vi "Enum Data Patch.vi"(7 "Ref":variant, 8 "error in (no error)":errorcluster, 11 "data in":variant) -> (0 "error out":errorcluster, 3 "data out":variant)   [LabVIEW 2017]
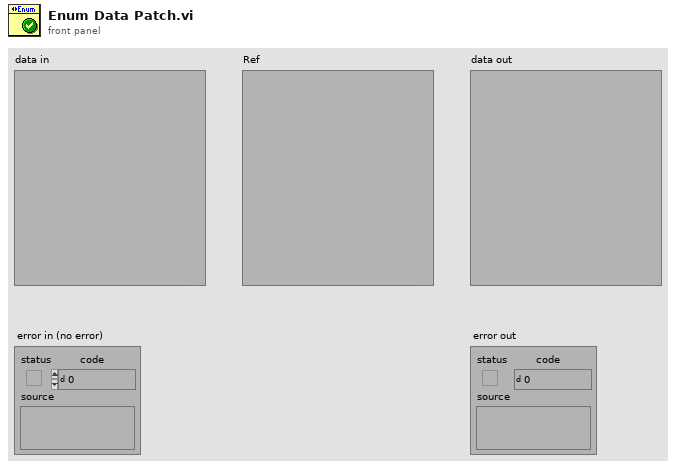
[diagram p1: front panel]
types:
  T1 = typedef "Type Descriptor Enumeration__ogtk.ctl" = enum8{"<Null>", "I8", "I16", "I32", "I64", "U8", "U16", "U32", "U64", "SGL", "DBL", "EXT", "CSG", "CDB", "CXT", "0x0F", "0x10", "0x11", "0x12", "0x13", "0x14", "Enum U8", "Enum U16", "Enum U32", "Enum U64", "SGL PQ", "DBL PQ", "EXT PQ", "CSG PQ", "CDB PQ", "CXT PQ", "0x1F", "0x20", "Boolean", "0x22", "0x23", "0x24", "0x25", "0x26", "0x27", "0x28", "0x29", "0x2A", "0x2B", "0x2C", "0x2D", "0x2E", "0x2F", "String", "0x31", "Path", "Pict", "0x34", "0x35", "0x36", "DAQ", "0x38", "0x39", "0x3A", "0x3B", "0x3C", "0x3D", "0x3E", "0x3F", "Array", "0x41", "0x42", "0x43", "0x44", "0x45", "0x46", "0x47", "0x48", "0x49", "0x4A", "0x4B", "0x4C", "0x4D", "0x4E", "0x4F", "Cluster", "0x51", "0x52", "Variant", "Waveform", "0x55", "0x56", "0x57", "0x58", "0x59", "0x5A", "0x5B", "0x5C", "0x5D", "0x5E", "0x5F", "0x60", "0x61", "0x62", "0x63", "0x64", "0x65", "0x66", "0x67", "0x68", "0x69", "0x6A", "0x6B", "0x6C", "0x6D", "0x6E", "0x6F", "Refnum"}
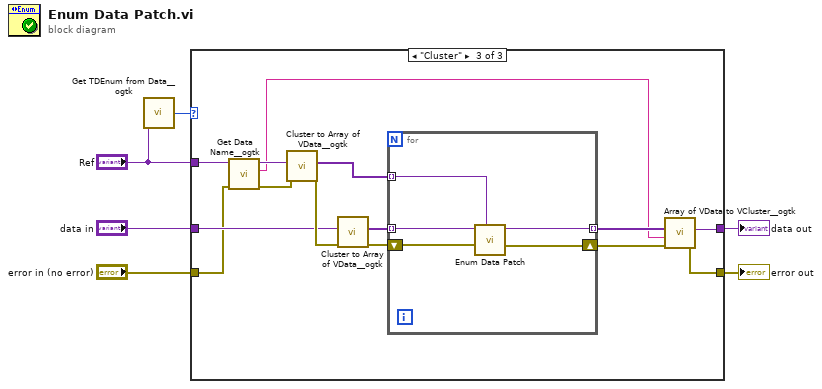
[diagram p0: block diagram]
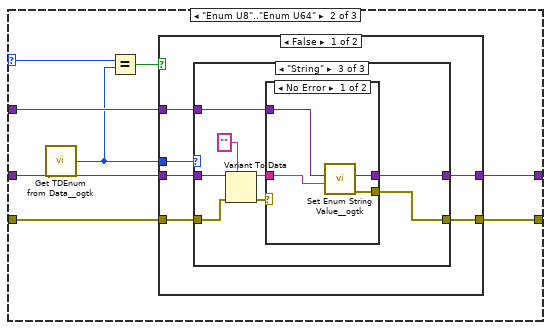
[diagram p3: hidden frame]
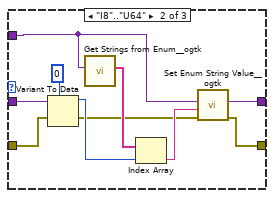
[diagram p5: hidden frame]
diagram:
  n1 = call <userlib>:"Get TDEnum from Data__ogtk.vi"("Data"="Ref") -> ("Type Descriptor Enumeration"=w6:T1)  [unwired: 4 in]
  n2 = case shown="\"Cluster\"" w6 {
    selector: w6 -> [_ w16 _]
    tunnel: [w8 w13 w63] -> w5
    tunnel: "data in" -> [w8 w10 w53]
    tunnel: "error in (no error)" -> [w7 w11 w52]
    tunnel: [w7 w12 w58] -> w2
    tunnel: "Ref" -> [_ w14 w55]
    frame Default {
    }
    frame "Enum U8".."Enum U64" {
      n3 = call <userlib>:"Get TDEnum from Data__ogtk.vi"("Data"=w10) -> ("Type Descriptor Enumeration"=w9:T1)  [unwired: 4 in]
      n4 = Equal?(x=w16, y=w9) -> (x = y?=w15:bool)
      n5 = case shown="False" w15 {
        tunnel: w14 -> [w21 _]
        tunnel: [w19 w48] -> w13
        tunnel: [w18 w49] -> w12
        tunnel: w11 -> [w17 w49]
        tunnel: w10 -> [w20 w48]
        tunnel: w9 -> [w22 _]
        frame False {
          n6 = case shown="\"String\"" w22 {
            tunnel: w21 -> [w24 w32 w41]
            tunnel: w20 -> [_ w34 w40]
            tunnel: [w24 w28 w42] -> w19
            tunnel: [w23 w26 w37] -> w18
            tunnel: w17 -> [w23 w25 w36]
            frame "<Null>", Default {
            }
            frame "I8".."U64" {
              n7 = Variant To Data(error in=w25, type=i64 0, Variant=w34) -> (data=w30:i64, error out=w27:errorcluster)
              n8 = call <userlib>:"Get Strings from Enum__ogtk.vi"("Enum"=w32) -> ("Enum Strings"=w31:string[])  [unwired: 7 in, 3 out]
              n9 = Index Array(array=w31, index=w30) -> (element=w29:string)
              n10 = call <userlib>:"Set Enum String Value__ogtk.vi"("error in (no error)"=w27, "String Value"=w29, "Default Enum Value"=w32) -> ("error out"=w26:errorcluster, "Enum"=w28:variant)  [unwired: 7 in]
            }
            frame "String" {
              n11 = Variant To Data(error in=w36, type="", Variant=w40) -> (data=w38:string, error out=w35:errorcluster)
              n12 = case shown="No Error" w35 {
                tunnel: [w46 w47] -> w42
                tunnel: w41 -> [w45 w47]
                tunnel: w38 -> [w44 _]
                tunnel: [w43 _] -> w37
                frame No Error {
                  n13 = call <userlib>:"Set Enum String Value__ogtk.vi"("String Value"=w44, "Default Enum Value"=w45) -> ("error out"=w43:errorcluster, "Enum"=w46:variant)  [unwired: 8 in]
                }
                frame Error {
                }
              }
            }
          }
        }
        frame True {
        }
      }
    }
    frame "Cluster" {
      n14 = call <userlib>:"Get Data Name__ogtk.vi"("error in (no error)"=w52, "Data"=w55) -> ("error out"=w51:errorcluster, "Data Name"=w50:string, "Data dup"=w54:variant)  [unwired: 7 in]
      n15 = call <userlib>:"Cluster to Array of VData__ogtk.vi"("error in (no error)"=w51, "Cluster"=w54) -> ("error out"=w56:errorcluster, "Array of VData"=w57:variant[])  [unwired: 8 in]
      n16 = call <userlib>:"Cluster to Array of VData__ogtk.vi"("error in (no error)"=w56, "Cluster"=w53) -> ("error out"=w60:errorcluster, "Array of VData"=w62:variant[])  [unwired: 8 in]
      n17 = for {
        tunnel: w62 -> [w68] mode=indexing
        tunnel: [w67] -> w61 mode=indexing
        shift-right: [w65] -> w59
        shift-left: w60 -> [w66]
        tunnel: w57 -> [w64] mode=indexing
        n18 = call "Enum Data Patch.vi"("Ref"=w64, "error in (no error)"=w66, "data in"=w68) -> ("error out"=w65:errorcluster, "data out"=w67:variant)  [unwired: 7 in]
      }
      n19 = call <userlib>:"Array of VData to VCluster__ogtk.vi"("error in (no error)"=w59, "Cluster Name"=w50, "Array"=w61) -> ("error out"=w58:errorcluster, "VCluster"=w63:variant)  [unwired: 7 in]
    }
  }
  "data out" <- w5
  "error out" <- w2
